vi "DAQ_compare_illumination_controls_clusters.vi"(2 "Illumination controls OLD":T1 {"641" min=0.0 max=100.0 step=0.10000000149011612 scale=0.0..100.0; "561" min=0.0 max=100.0 step=0.10000000149011612 scale=0.0..100.0; "405" min=0.0 max=100.0 step=0.10000000149011612 scale=0.0..100.0; "488" min=0.0 max=100.0 step=0.10000000149011612 scale=0.0..100.0; "BF" min=0.0 max=100.0 step=0.1 scale=0.0..100.0}, 3 "Illumination controls NEW":T1 {"641" min=0.0 max=100.0 step=0.10000000149011612 scale=0.0..100.0; "561" min=0.0 max=100.0 step=0.10000000149011612 scale=0.0..100.0; "405" min=0.0 max=100.0 step=0.10000000149011612 scale=0.0..100.0; "488" min=0.0 max=100.0 step=0.10000000149011612 scale=0.0..100.0; "BF" min=0.0 max=100.0 step=0.1 scale=0.0..100.0}, 4 "error in":errorcluster) -> (0 "Array":i32[](array[numeric]), 1 "error out":errorcluster)   [LabVIEW 2015]
uses:
  CONTROLS/Illumination and filters.ctl
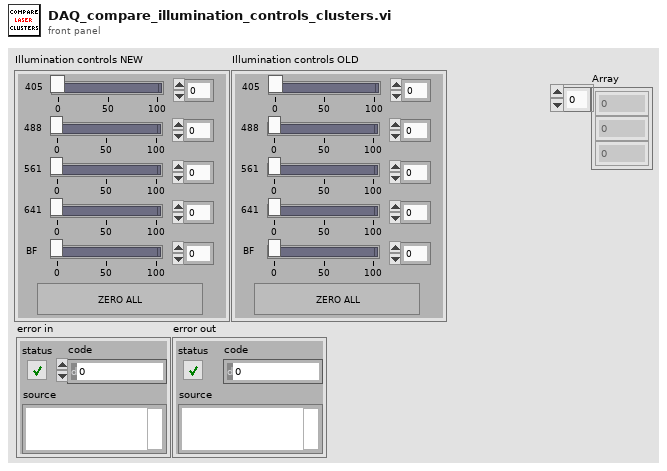
[diagram p1: front panel]
types:
  T1 = typedef "Illumination and filters.ctl" = cluster{"BF ":dbl, "641":dbl, "561":dbl, "488":dbl, "405":dbl, "ZERO ALL":bool}
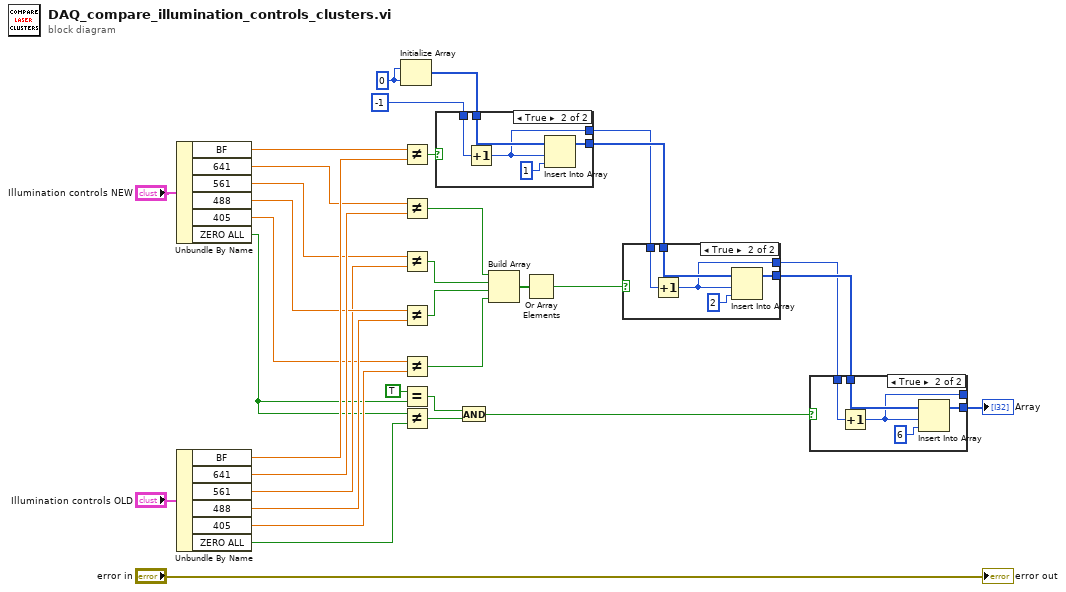
[diagram p0: block diagram]
diagram:
  w19 = 0 ("dimension size")
  n1 = Unbundle By Name("Illumination controls NEW") -> ("BF"=w32:dbl, "641"=w29:dbl, "561"=w27:dbl, "488"=w25:dbl, "405"=w21:dbl, "ZERO ALL"=w14:bool)
  n2 = Unbundle By Name("Illumination controls OLD") -> ("BF"=w31:dbl, "641"=w28:dbl, "561"=w24:dbl, "488"=w26:dbl, "405"=w23:dbl, "ZERO ALL"=w22:bool)
  n3 = Initialize Array(w19, w19) -> (w20:i32[])
  n4 = Not Equal?(x=w32, y=w31) -> (x != y?=w30:bool)
  n5 = Not Equal?(x=w29, y=w28) -> (x != y?=w10:bool)
  n6 = Not Equal?(x=w27, y=w24) -> (x != y?=w9:bool)
  n7 = Not Equal?(x=w25, y=w26) -> (x != y?=w8:bool)
  n8 = Not Equal?(x=w21, y=w23) -> (x != y?=w7:bool)
  n9 = Equal?(x=TRUE, y=w14) -> (x = y?=w12:bool)
  n10 = Not Equal?(x=w14, y=w22) -> (x != y?=w15:bool)
  n11 = case shown="True" w30 {
    tunnel: w20 -> [w36 w41]
    tunnel: -1 ("dimension size") -> [w35 w39]
    tunnel: [w36 w38] -> w4
    tunnel: [w35 w37] -> w3
    frame False {
    }
    frame True {
      n12 = Increment(x=w39) -> (x+1=w37:i32)
      n13 = Insert Into Array(array=w41, index=w37, new element=1 ("index")) -> (w38:i32[])
    }
  }
  n14 = And(x=w12, y=w15) -> (x .and. y?=w11:bool)
  n15 = Build Array(w10, w9, w8, w7) -> (w6:bool[])
  n16 = Or Array Elements(Boolean array=w6) -> (logical OR=w5:bool)
  n17 = case shown="True" w5 {
    tunnel: w4 -> [w43 w48]
    tunnel: w3 -> [w42 w46]
    tunnel: [w43 w45] -> w2
    tunnel: [w42 w44] -> w1
    frame False {
    }
    frame True {
      n18 = Increment(x=w46) -> (x+1=w44:i32)
      n19 = Insert Into Array(array=w48, index=w44, new element=2 ("index")) -> (w45:i32[])
    }
  }
  n20 = case shown="True" w11 {
    tunnel: w2 -> [w50 w55]
    tunnel: w1 -> [w49 w53]
    tunnel: [w50 w52] -> w16
    tunnel: [w49 w51] -> _
    frame False {
    }
    frame True {
      n21 = Increment(x=w53) -> (x+1=w51:i32)
      n22 = Insert Into Array(array=w55, index=w51, new element=6 ("index")) -> (w52:i32[])
    }
  }
  "Array" <- w16
  "error out" <- "error in"
